vi "Item_OnCommand.vi"(10 "Command ID":string, 11 "Object":T1) -> ()   [LabVIEW 2020, in "Project Provider.lvlib"]
uses:
  Project Provider.lvlib
  <resource>/Framework/Providers/API/ItemRef.ctl
panel:
  out "error out":errorcluster
  in  "error in":errorcluster
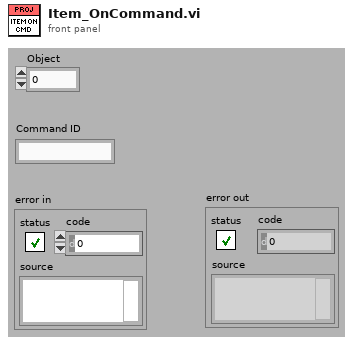
[diagram p1: front panel]
types:
  T1 = typedef "ItemRef.ctl" = u64
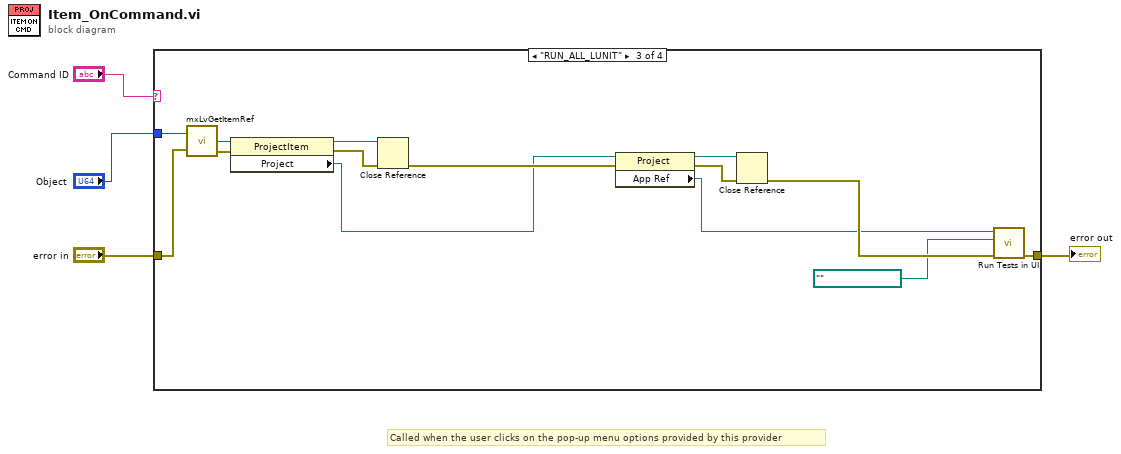
[diagram p0: block diagram]
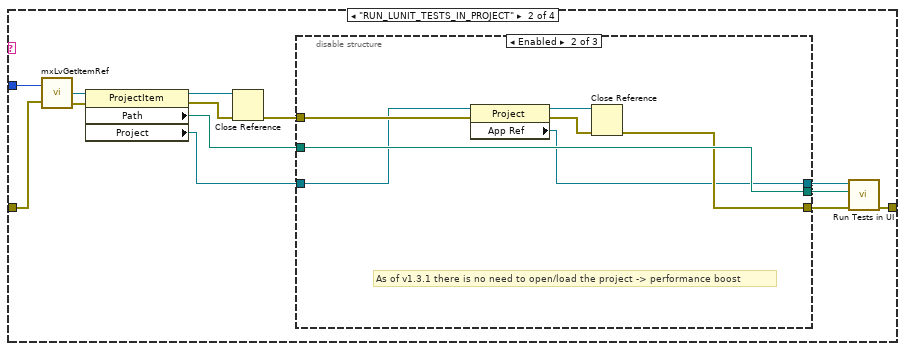
[diagram p3: hidden frame]
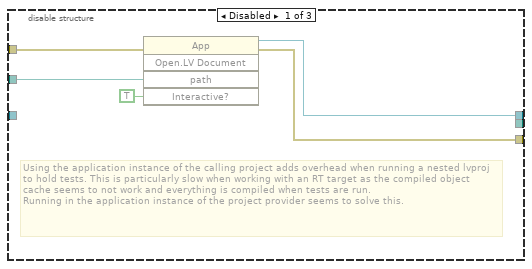
[diagram p4: hidden frame]
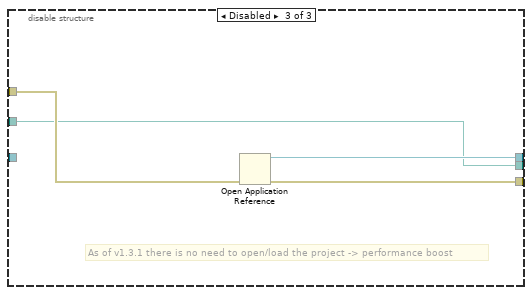
[diagram p5: hidden frame]
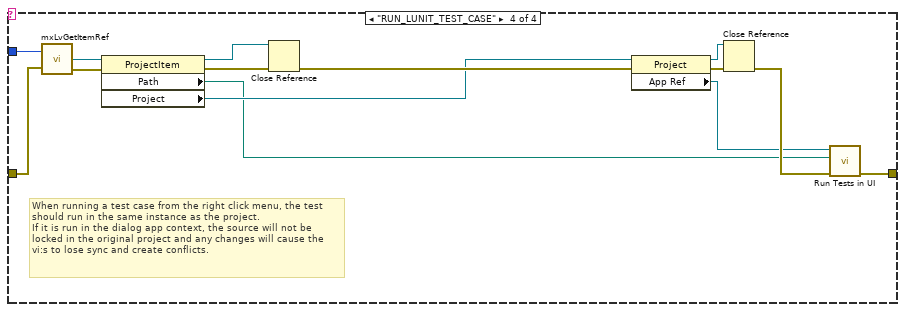
[diagram p6: hidden frame]
diagram:
  # "Called when the user clicks on the pop-up menu options provided by this provider"
  n1 = case shown="\"RUN_ALL_LUNIT\"" "Command ID" {
    tunnel: "error in" -> [w5 w17 w47 w61]
    tunnel: [w5 w11 w41 w56] -> w2
    tunnel: "Object" -> [_ w18 w48 w62]
    frame Default {
    }
    frame "RUN_LUNIT_TESTS_IN_PROJECT" {
      n2 = call <resource>:"mxLvGetItemRef.vi"("Item"=w18, "error in"=w17) -> ("Item Refnum"=w16:refnum<vi>, "error out"=w13:errorcluster)  [unwired: 1 out]
      n3 = property class="ProjectItem"(reference=w16, error in=w13) -> (reference out=w14:refnum<vi>, error out=w15:errorcluster, "Path"=w9:path, "Project"=w6:refnum<vi>)
      n4 = Close Reference(reference=w14, error in (no error)=w15) -> (error out=w12:errorcluster)
      n5 = disable-structure shown="Enabled" {
        disable-tunnel: w12 -> [w23 w27 w32]
        disable-tunnel: [w22 w26 w33] -> w10
        disable-tunnel: w9 -> [w21 w30 w31]
        disable-tunnel: [w19 w24 w34] -> w8
        disable-tunnel: [_ w30 w31] -> w7
        disable-tunnel: w6 -> [_ w25 _]
        frame Disabled {
          # "Using the application instance of the calling project adds overhead when running a nested lvproj to hold tests. This is particularly slow when working with an RT target as the compiled object cache seems to not work and everything is compiled when tests are run.\nRunning in the application instance of the project provider seems to solve this."
          n6 = invoke class="App" method="Open.LV Document"(error in=w23, "path"=w21, "Interactive?"=TRUE) -> (reference out=w19:refnum<vi>, error out=w22:errorcluster)  [unwired: 2 in, 3 out]
        }
        frame Enabled {
          # "As of v1.3.1 there is no need to open/load the project -> performance boost"
          n7 = property class="Project"(reference=w25, error in=w27) -> (reference out=w29:refnum<vi>, error out=w28:errorcluster, "App Ref"=w24:refnum<vi>)
          n8 = Close Reference(reference=w29, error in (no error)=w28) -> (error out=w26:errorcluster)
        }
        frame Disabled {
          # "As of v1.3.1 there is no need to open/load the project -> performance boost"
          n9 = Open Application Reference(8:w32) -> (0:w33:errorcluster, 3:w34:refnum<vi>)  [unwired: 3 in]
        }
      }
      n10 = call "Run Tests in UI.vi"("error in (no error)"=w10, "Path"=w7, "Application"=w8) -> ("error out"=w11:errorcluster)  [unwired: 8 in]
    }
    frame "RUN_ALL_LUNIT" {
      n11 = call <resource>:"mxLvGetItemRef.vi"("Item"=w48, "error in"=w47) -> ("Item Refnum"=w46:refnum<vi>, "error out"=w43:errorcluster)  [unwired: 1 out]
      n12 = property class="ProjectItem"(reference=w46, error in=w43) -> (reference out=w44:refnum<vi>, error out=w45:errorcluster, "Project"=w38:refnum<vi>)
      n13 = Close Reference(reference=w44, error in (no error)=w45) -> (error out=w42:errorcluster)
      n14 = property class="Project"(reference=w38, error in=w42) -> (reference out=w37:refnum<vi>, error out=w36:errorcluster, "App Ref"=w39:refnum<vi>)
      n15 = Close Reference(reference=w37, error in (no error)=w36) -> (error out=w40:errorcluster)
      n16 = call "Run Tests in UI.vi"("error in (no error)"=w40, "Path"=path "", "Application"=w39) -> ("error out"=w41:errorcluster)  [unwired: 8 in]
    }
    frame "RUN_LUNIT_TEST_CASE" {
      # "When running a test case from the right click menu, the test should run in the same instance as the project.\nIf it is run in the dialog app context, the source will not be locked in the original project and any changes will cause the vi:s to lose sync and create conflicts."
      n17 = call <resource>:"mxLvGetItemRef.vi"("Item"=w62, "error in"=w61) -> ("Item Refnum"=w60:refnum<vi>, "error out"=w57:errorcluster)  [unwired: 1 out]
      n18 = property class="ProjectItem"(reference=w60, error in=w57) -> (reference out=w58:refnum<vi>, error out=w59:errorcluster, "Path"=w51:path, "Project"=w52:refnum<vi>)
      n19 = Close Reference(reference=w58, error in (no error)=w59) -> (error out=w54:errorcluster)
      n20 = property class="Project"(reference=w52, error in=w54) -> (reference out=w50:refnum<vi>, error out=w49:errorcluster, "App Ref"=w53:refnum<vi>)
      n21 = Close Reference(reference=w50, error in (no error)=w49) -> (error out=w55:errorcluster)
      n22 = call "Run Tests in UI.vi"("error in (no error)"=w55, "Path"=w51, "Application"=w53) -> ("error out"=w56:errorcluster)  [unwired: 8 in]
    }
  }
  "error out" <- w2
